vi "列表框写列数组.vi"(8 "新元素/子数组":string[](array[string]), 9 "列":i32, 11 "引用":refnum<vi>) -> ()   [LabVIEW 2016]
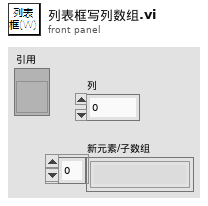
[diagram p1: front panel]
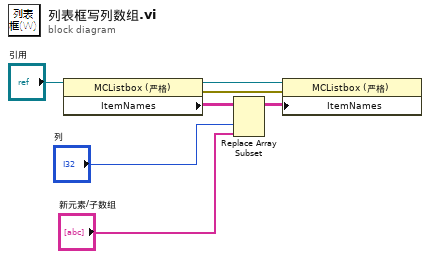
[diagram p0: block diagram]
diagram:
  n1 = property class="MCListbox (严格)"(reference="引用") -> (reference out=w3:refnum<vi>, error out=w2:errorcluster, "ItemNames"=w6:string[][])  [unwired: 1 in]
  n2 = Replace Array Subset(array=w6, new element="新元素/子数组", index (col)="列") -> (w1:string[][])  [unwired: 1 in]
  n3 = property class="MCListbox (严格)"(reference=w3, error in=w2, "ItemNames"=w1) -> ()  [unwired: 2 out]
